vi "convertor imagine2.vi"() -> ()   [LabVIEW 2024]
uses:
  <vilib>/vision/NI_Vision_Development_Module.lvlib
panel:
  out "stripped path":path
  out "Image 2":T1(plugin-control)
  out "appended path":path
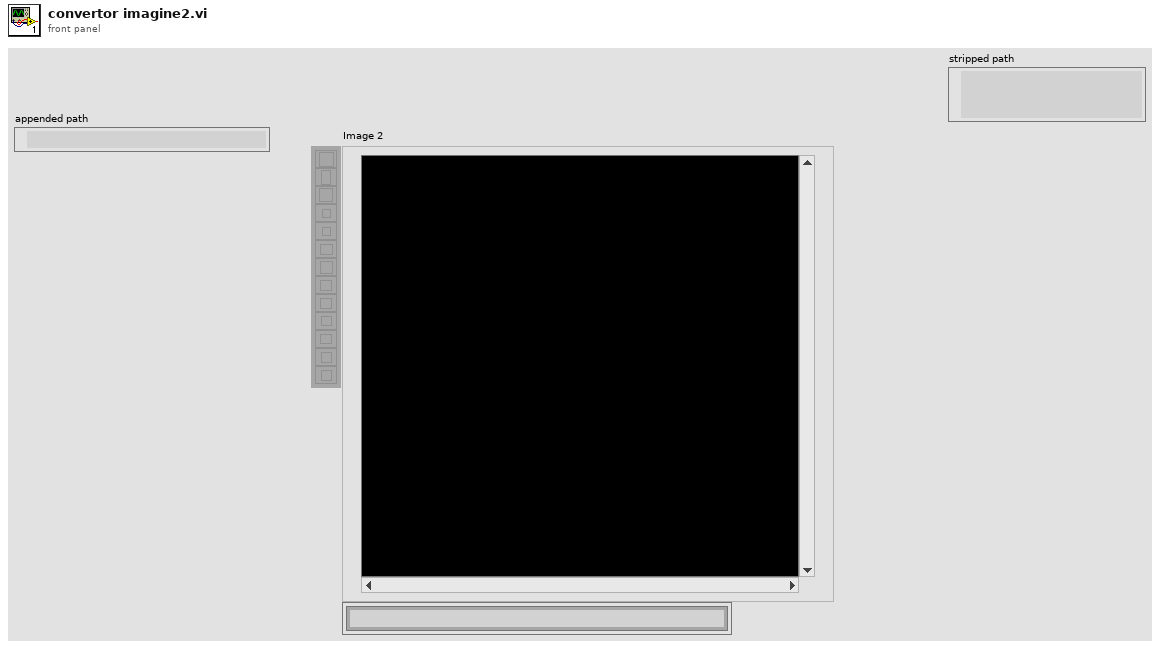
[diagram p1: front panel]
types:
  T1 = typedef "IMAQ Image.ctl" = refnum<image>
  T2 = typedef "Color (U64)" = cluster{"Plane 3 (Blue)":u16, "Plane 2 (Green)":u16, "Plane 1 (Red)":u16, "Plane 4 (alpha)":u16}
  T3 = typedef "Image Type" = u32
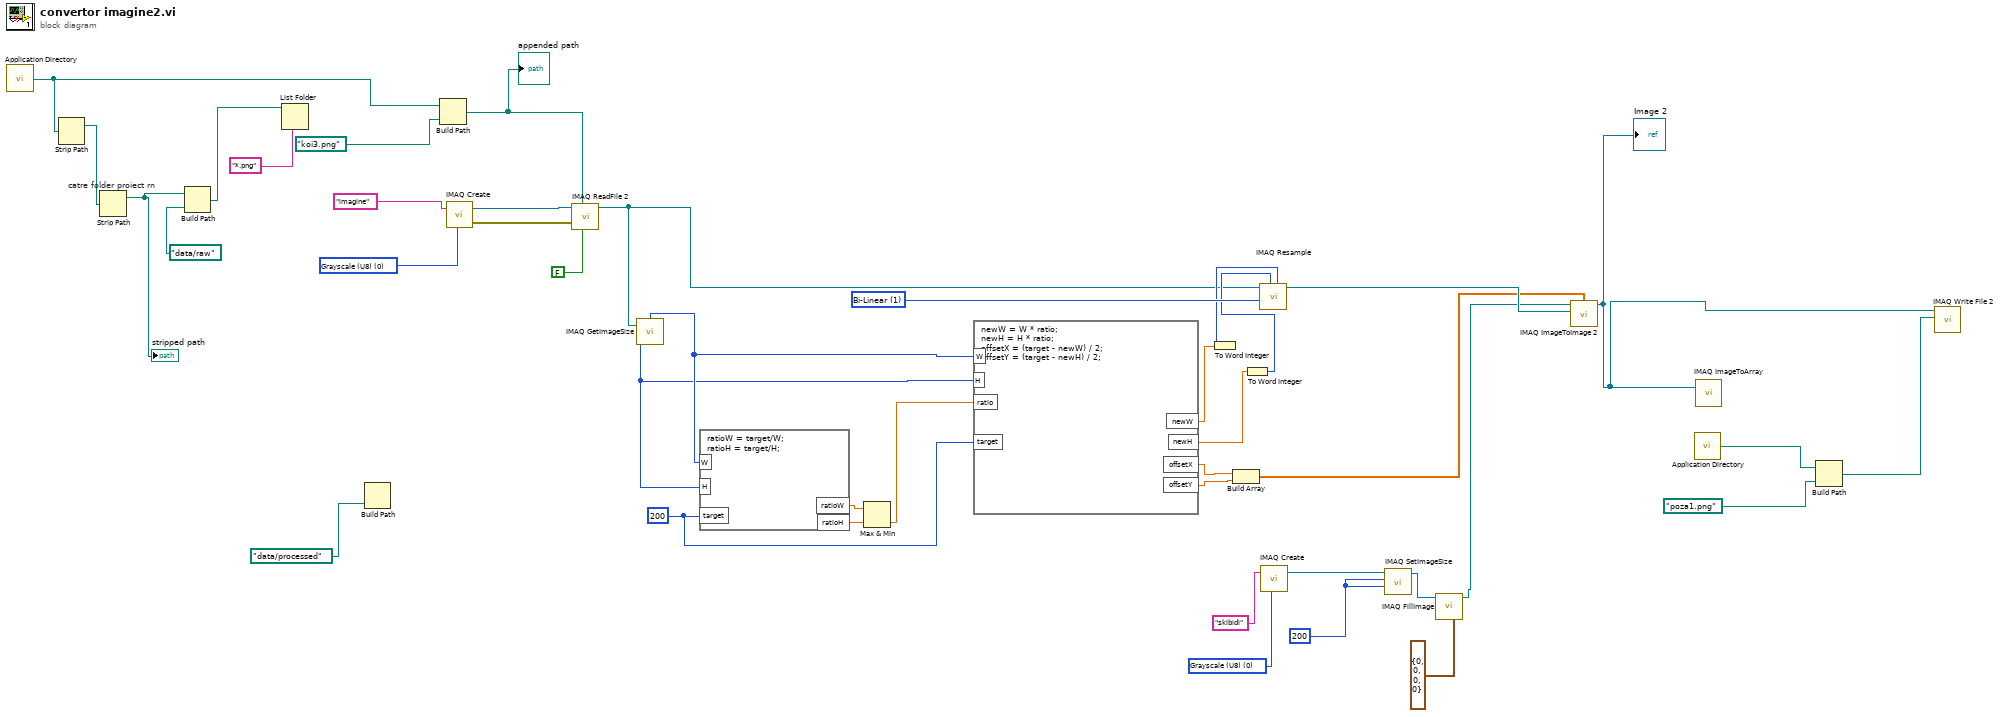
[diagram p0: block diagram]
diagram:
  w21 = 200 ("Y Resolution")
  w23 = T3 0 items=["Grayscale (U8)", "Grayscale (I16)", "Grayscale (SGL)", "Complex (CSG)", "RGB (U32)", "HSL (U32)", "RGB (U64)", "Grayscale (U16)"] ("Image Type")
  w28 = u32 1 items=["Zero Order", "Bi-Linear", "Quadratic", "Cubic Spline"] ("Interpolation Type")
  w29 = 200
  w40 = T3 0 items=["Grayscale (U8)", "Grayscale (I16)", "Grayscale (SGL)", "Complex (CSG)", "RGB (U32)", "HSL (U32)", "RGB (U64)", "Grayscale (U16)"] ("Image Type")
  n1 = call <vilib>:"Application Directory.vi"() -> ("Application Directory"=w3:path)
  n2 = Strip Path(path=w3) -> (stripped path=w6:path)  [unwired: 1 out]
  n3 = Strip Path "catre folder proiect rn"(path=w6) -> (stripped path=w5:path)  [unwired: 1 out]
  "stripped path" <- w5
  n4 = Build Path(base path=w5, name or relative path=path "data/raw") -> (appended path=w2:path)
  n5 = List Folder(path=w2, pattern="*.png") -> ()  [unwired: 2 in, 4 out]
  n6 = Build Path(name or relative path=path "data/processed") -> ()  [unwired: 1 in, 1 out]
  n7 = Build Path(base path=w3, name or relative path=path "koi3.png" ("File Path")) -> (appended path=w37:path)
  "appended path" <- w37
  n8 = call "IMAQ Create"("Image Name"="imagine", "Image Type"=w40) -> ("New Image"=w35:T1, "error out"=w39:errorcluster)  [unwired: 3 in]
  n9 = call "IMAQ ReadFile 2"("Use File Path Image Type"=FALSE, "File Path"=w37, "error in (no error)"=w39, "Image"=w35) -> ("Image Out"=w13:T1)  [unwired: 3 in, 4 out]
  n10 = call "IMAQ GetImageSize"("Image"=w13) -> ("Y Resolution"=w30:i32, "X Resolution"=w31:i32)  [unwired: 3 in, 1 out]
  n11 = formula code="ratioW = target/W;\nratioH = target/H;"("W"=w31, "H"=w30, "target"=w29) -> ("ratioW"=w34:dbl, "ratioH"=w33:dbl)
  n12 = Max & Min(x=w34, y=w33) -> (min(x,y)=w32:dbl)  [unwired: 1 out]
  n13 = formula code="newW = W * ratio;\nnewH = H * ratio;\noffsetX = (target - newW) / 2;\noffsetY = (target - newH) / 2;"("ratio"=w32, "W"=w31, "H"=w30, "target"=w29) -> ("newW"=w25:dbl, "newH"=w27:dbl, "offsetX"=w14:dbl, "offsetY"=w15:dbl)
  n14 = To Word Integer(number=w25) -> (16bit integer=w24:i16)
  n15 = Build Array(w14, w15) -> (w12:dbl[])
  n16 = To Word Integer(number=w27) -> (16bit integer=w26:i16)
  n17 = call "IMAQ Resample"("X Resolution"=w24, "Y Resolution"=w26, "Interpolation Type"=w28, "Image Src"=w13) -> ("Image Dst Out"=w19:T1)  [unwired: 6 in, 1 out]
  n18 = call "IMAQ Create"("Image Name"="skibidi", "Image Type"=w23) -> ("New Image"=w22:T1)  [unwired: 3 in, 1 out]
  n19 = call "IMAQ SetImageSize"("Y Resolution"=w21, "X Resolution"=w21, "Image"=w22) -> ("Image Out"=w17:T1)  [unwired: 2 in, 1 out]
  n20 = call "IMAQ FillImage"("Color (U64)"=T2 {"Plane 3 (Blue)"=0, "Plane 2 (Green)"=0, "Plane 1 (Red)"=0, "Plane 4 (alpha)"=0}, "Image"=w17) -> ("Image Out"=w16:T1)  [unwired: 8 in, 1 out]
  n21 = call "IMAQ ImageToImage 2"("Offset Left/Top"=w12, "Image Src (Small)"=w19, "Image Src (Large)"=w16) -> ("Image Dst Out"=w11:T1)  [unwired: 7 in, 1 out]
  "Image 2" <- w11
  n22 = call <vilib>:"Application Directory.vi"() -> ("Application Directory"=w9:path)
  n23 = call "IMAQ ImageToArray"("Image"=w11) -> ()  [unwired: 3 in, 5 out]
  n24 = Build Path(base path=w9, name or relative path=path "poza1.png" ("File Path")) -> (appended path=w8:path)
  n25 = call-poly "IMAQ Write File 2"("File Path"=w8, "Image"=w11) -> ()  [unwired: 8 in, 2 out]
